vi "RS232Request.vi"(1 "InputFIFO":refnum<k21>="DisplacementTxFIFO") -> ()   [LabVIEW 2016]
uses:
  <vilib>/rvi/DataTransferAndStorage/Container/Common/niFpgaContainerExecOnDevCompGetState.vi
  <vilib>/rvi/Emulation/niFpgaEmulationIsFPGAContextNoSignature.vi
  <vilib>/rvi/Emulation/niFpgaSctlEmulationGetInTimedLoop.vi
  <vilib>/rvi/errors/niFpgaSetErrorForExecOnDevCompSimple.vi
  <vilib>/rvi/eio/common/nirviEmuReportErrorAndStop.vi
  <vilib>/rvi/DataTransferAndStorage/Container/Common/niFpgaContainerGetUniqueNameForEmu.vi
  <vilib>/rvi/FIFO/Fifo_Resource/nirvififoEmulationSetSize.vi
  <vilib>/rvi/FIFO/Fifo_Resource/nirviFifoEmulationQueueMgr.vi
  <instcachedir>/0/nirviFifoEmulationQueueMgr_E5CAEC123FF24DC58D834DCA3CDAA9B5.lvgen/nirviFifoEmulationQueueMgr_E5CAEC123FF24DC58D834DCA3CDAA9B5_009.vi
  <vilib>/rvi/FIFO/Fifo_Resource/nirvififoEmulationDetermineInputValidOut.vi
  <vilib>/rvi/FIFO/Fifo_Resource/nirvififoEmulationCreateLock.vi
  <vilib>/rvi/Emulation/niFpgaProcessEmulError.vi
  <vilib>/rvi/FIFO/Fifo_Resource/nirvififoEmulationObtainLock.vi
  <vilib>/rvi/FIFO/Fifo_Resource/nirvififoEmulationReleaseLock.vi
  <vilib>/rvi/occurrence/nirviWaitOnOccurrenceBase.vi
  <vilib>/rvi/errors/nirviReportUnexpectedCaseInternalError.vi
  <vilib>/rvi/errors/nirviReportUnexpectedCaseInternalError (U32).vi
  <vilib>/Utility/error.llb/Clear Errors.vi
  <vilib>/rvi/interface/RandomDataEmulation/niFpgaRandomDataHandleErrors.vi
  <vilib>/rvi/DataTransferAndStorage/Container/XNode/niFpgaContainer.xnode
  <vilib>/rvi/FIFO/Fifo_Resource/niFpgaFifoEmulationRefIn.vi
  Common_FPGA_FIFO/FPGAFIFO.lvlib
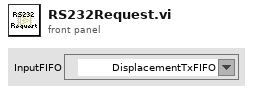
[diagram p1: front panel]
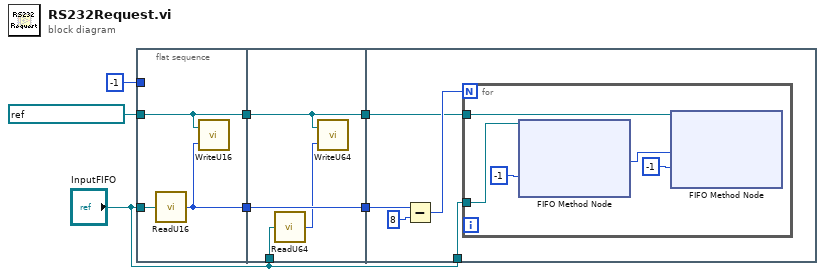
[diagram p0: block diagram]
diagram:
  n1 = flat-sequence {
    tunnel: "InputFIFO" -> [w10]
    tunnel: -1 ("Timeout") -> [_]
    tunnel: [w9] -> w3
    tunnel: refnum<k21> "U8ResponseFIFO" ("FIFO") -> [w8]
    tunnel: [w8] -> w1
    tunnel: [w13] -> w7
    tunnel: "InputFIFO" -> [w14]
    tunnel: [w11] -> w5
    tunnel: w3 -> [w13]
    tunnel: w1 -> [w11]
    tunnel: w7 -> [w19]
    tunnel: "InputFIFO" -> [w16]
    tunnel: w5 -> [w15]
    frame #0 {
      n2 = call "ReadU16.vi"("FIFO"=w10) -> ("U16"=w9:u16)
      n3 = call "WriteU16.vi"("U16"=w9, "FIFO"=w8) -> ()  [unwired: 1 in]
    }
    frame #1 {
      n4 = call "ReadU64.vi"("FIFO"=w14) -> ("U64"=w12:u64)
      n5 = call "WriteU64.vi"("U64"=w12, "FIFO"=w11) -> ()  [unwired: 1 in]
    }
    frame #2 {
      n6 = Subtract(x=w19, y=u16 8) -> (x-y=w17:u16)
      n7 = for {
        N: w17 -> [_]
        tunnel: w16 -> [w21]
        tunnel: w15 -> [w20]
        n8 = xnode ("FIFO Method Node")("Timeout"=-1, "FIFO In"=w21) -> ("Element"=w22:u8)  [unwired: 2 out]
        n9 = xnode ("FIFO Method Node")("Element"=w22, "Timeout"=-1, "FIFO In"=w20) -> ()  [unwired: 2 out]
      }
    }
  }
